vi "1-N随机排列自然数（数组重排）.vi"(1 "Num (100)":i32=100) -> (0 "1-N":i32[](array[numeric]))   [LabVIEW 2012]
doc: "功能：\n\n产生1-N自然数随机排列的数组。\n\n\n基本算法：\n\n通过产生0-N-1个白噪声（均匀分布随机数），利用信号函数选板的重排数组函数，得到0-N-1的随机排列。\n\ncsxcs_366创建"
uses:
  <vilib>/Analysis/1siggen.llb/Riffle Array (DBL) (obs 2012).vi
  <vilib>/Analysis/NI_AALBase.lvlib
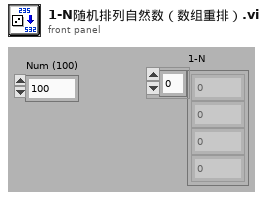
[diagram p1: front panel]
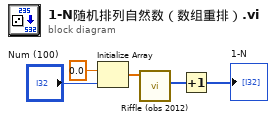
[diagram p0: block diagram]
diagram:
  n1 = Initialize Array(0.0 ("元素"), "Num (100)") -> (w5:dbl[])
  n2 = call-poly <vilib>:"Riffle (obs 2012).vi"("X"=w5) -> ("Riffled Index"=w2:i32[])  [unwired: 8 in, 2 out]
  n3 = Increment(x=w2) -> (x+1=→"1-N":i32[])
